vi "FPGA Host-integration mode.vi"() -> ()   [LabVIEW 2015]
uses:
  <vilib>/eio/EIONode/EIONode.xnode
  <vilib>/rvi/eio/common/nirviEmuTemplateMethod_errors.vi
  Globals/Global_Sample per Frame.vi
  Globals/Global Variable_Pixel Clock.vi
panel:
  in  "Number of frames":i32
  out "Samples acquired":u32
  out "Samples per frame_Global":u32
  out "Frame waveform output finish?":bool
  out "Frame acquisition finish?":bool
  out "SubVi Indicator":i32
  out "image data address indicator":u32
  out "Data indicator":u32
  out "Address counter":u32
  out "Pixel clock_indicator":bool
  out "Frame address_indicator":u32
  out "Averaged image displayed? _indicator":bool
  out "Scanning?":bool
  out "loop count":i32
  out "Display_frames done":i32
  out "Averaged data address":u32
  out "Frame imaging data averaged?":bool
  out "Averaged image displayed?":bool
  in  "Kalman gain":fxp<+,16,1>=0.1015625
  in  "Filter gain":fxp<+,16,0>=0.8000030517578125
  in  "Ready to Scan":bool
  out "Pixel clock (Indicator)":bool
  out "Image averaging done?":bool
  in  "Samples per frame control":u32=262144
  out "Data":u32
  out "Galvo signal readed":u32
  out "Request address":u32
  out "Line clock":bool
  in  "Pixel clock_pulse width(tick)":i32
  in  "Resolution":i32
  in  "Pixel pulse_initial delay":i32
  in  "Frame retrace time":u32 caption="Frame retrace time (ms)"
  in  "Num of undershoot":i32
  in  "Elements per line":i32
  in  "Num of elements":u32
  in  "Pixel time (tick)":i32
  out "Write DRAM done?":bool
  in  "Total elements":u32
  out "Frame Galvo signal write done?":bool
  in  "max addr":u32=1024
  in  "Write DRAM enable?":bool
  in  "Write Frame Galvo signal?":bool
  # "Waveform Data Loading"
  # "Photon Counting"
  # "Waveform Generation"
  # "Controller"
  # "Indicator"
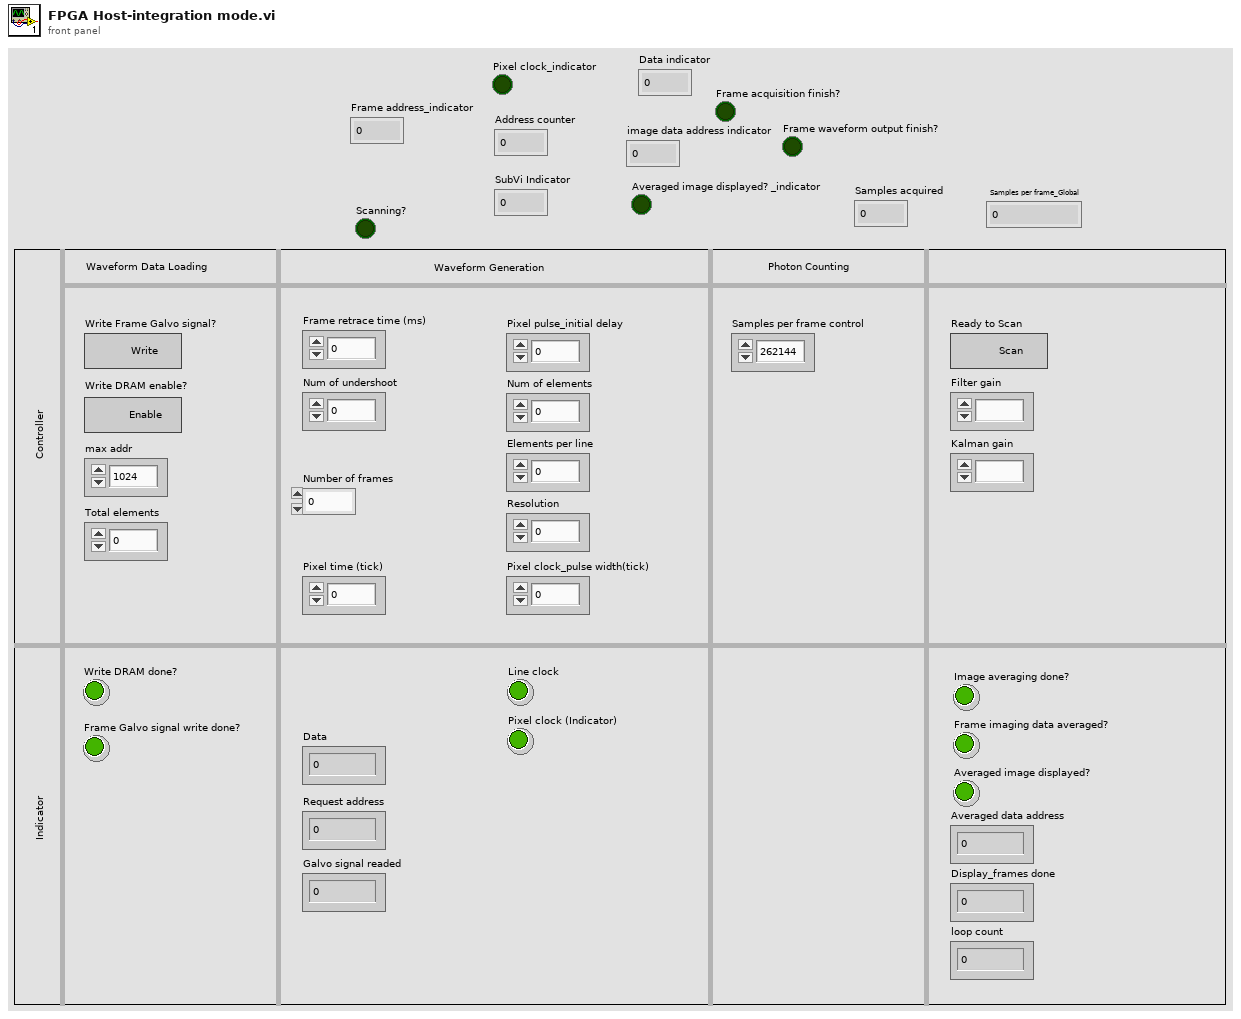
[diagram p1: front panel]
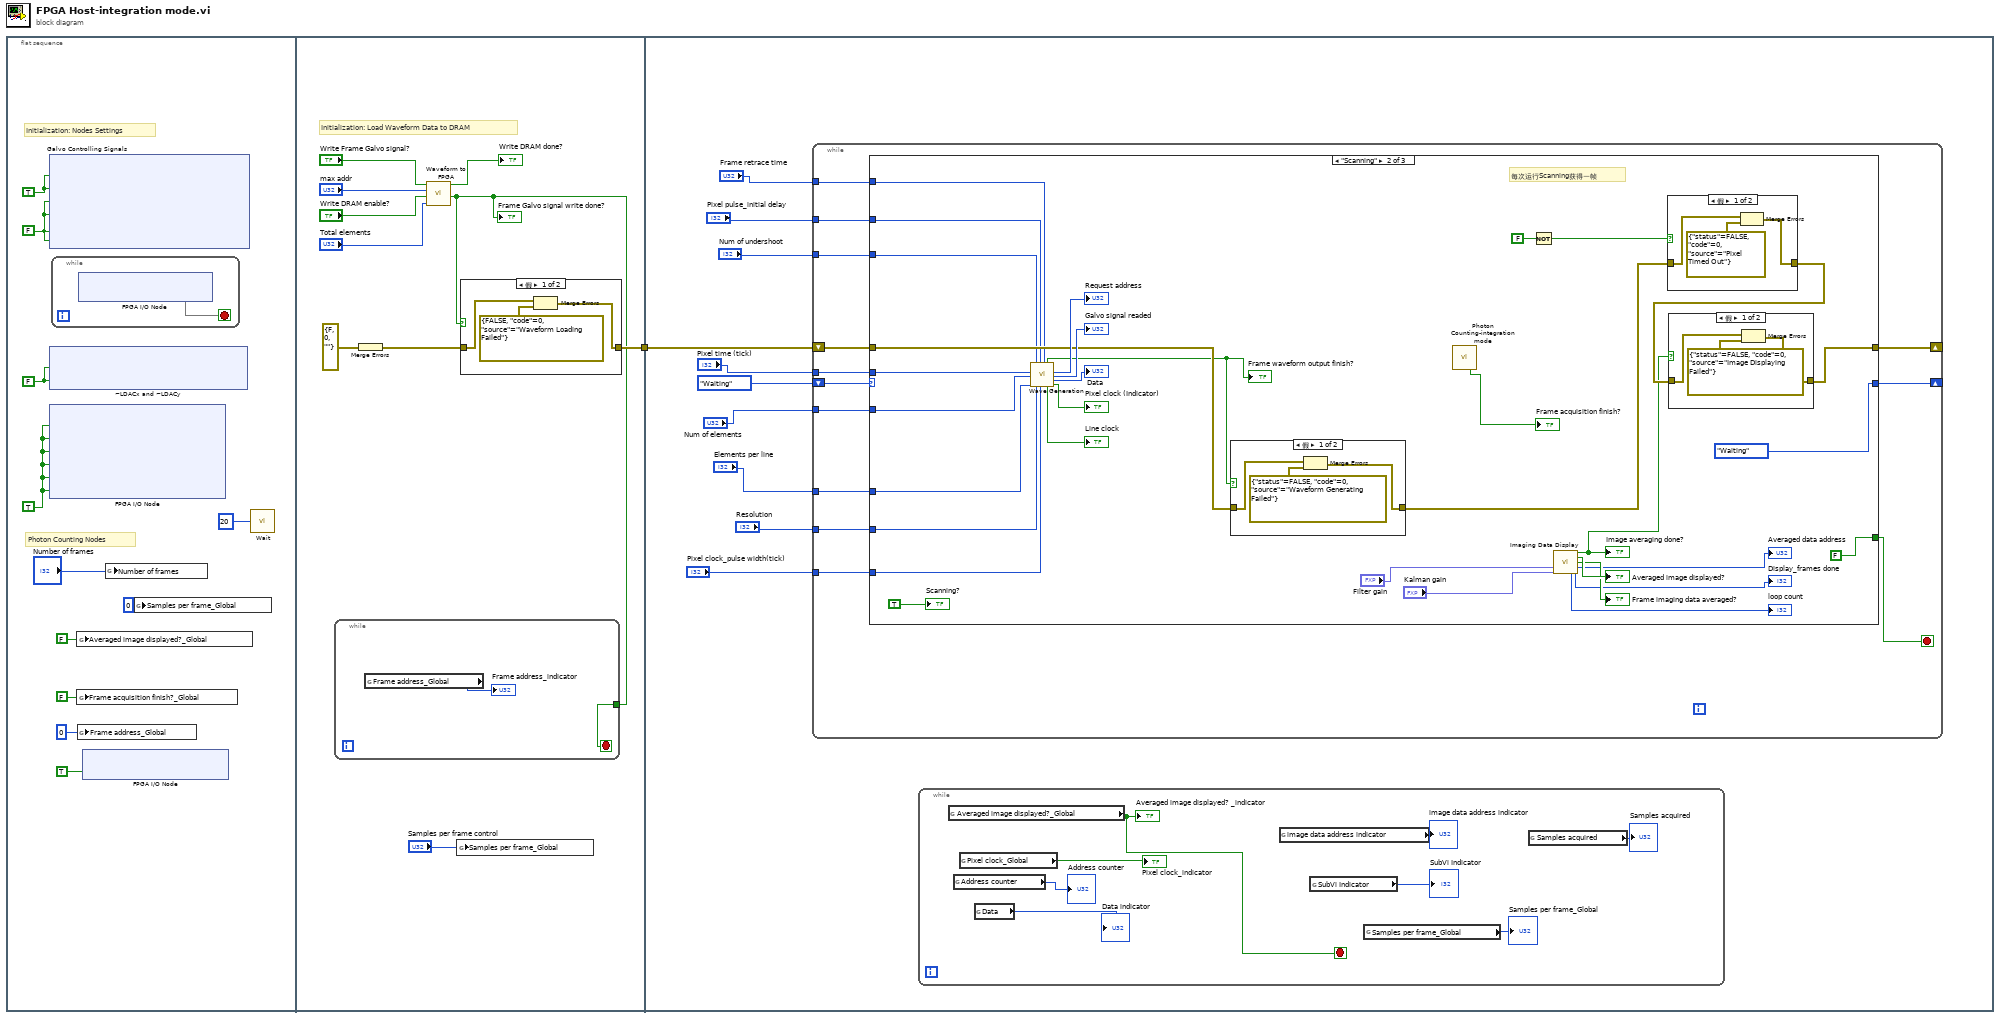
[diagram p0: block diagram]
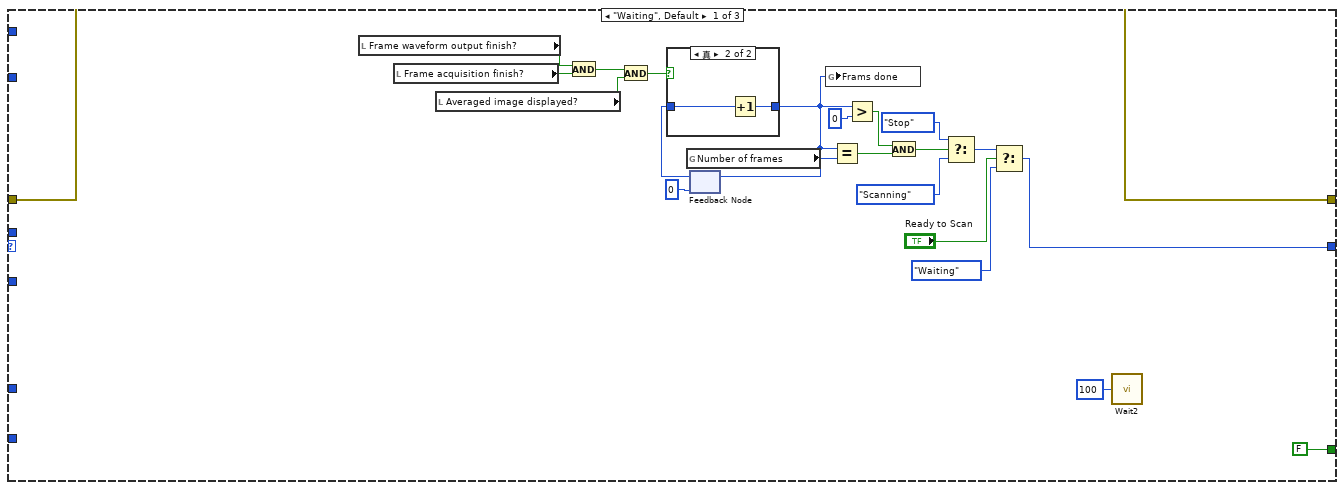
[diagram p3: hidden frame]
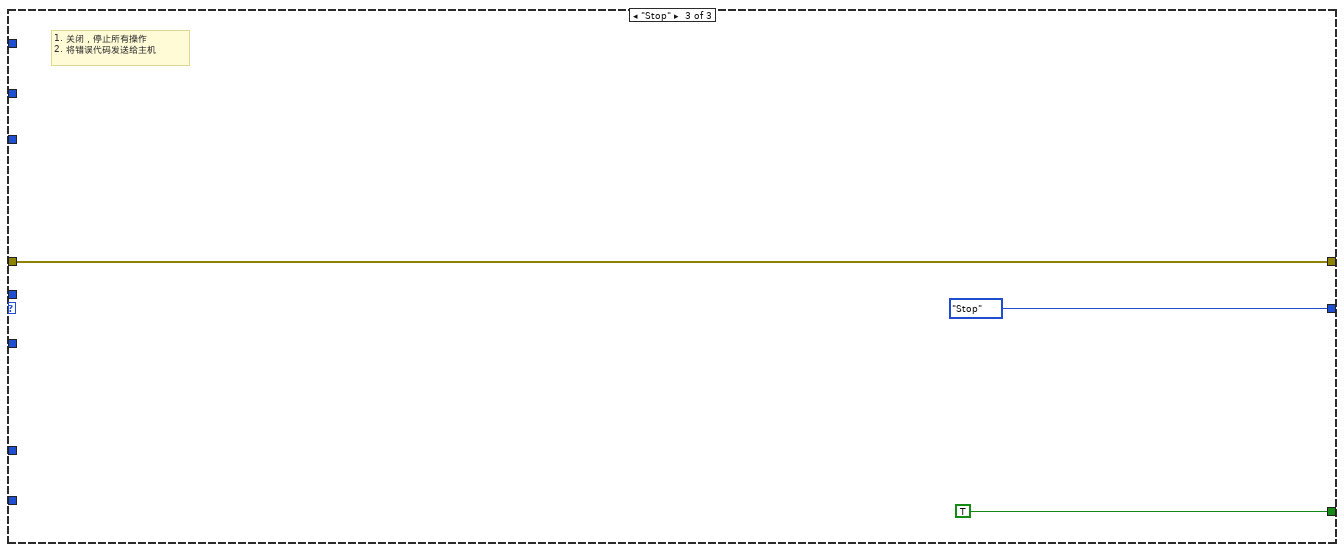
[diagram p8: hidden frame]
diagram:
  n1 = flat-sequence {
    tunnel: [w16] -> w1
    tunnel: w1 -> [w38]
    frame #0 {
      w9 = TRUE ("IO Module\\DDCA_DIO8-15_WE")
      w10 = FALSE ("_LDACx")
      w11 = FALSE ("_CSx")
      w12 = TRUE ("_CLRx")
      # "Photon Counting Nodes"
      # "Initialization: Nodes Settings"
      n2 = xnode "Galvo Controlling Signals"("IO Module\\CLRx(DDCB_DIO0_WRITE)"=w12, "IO Module\\CLRy(DDCB_DIO1_WRITE)"=w12, "IO Module\\CSx(DDCB_DIO2_WRITE)"=w11, "IO Module\\CSy(DDCB_DIO3_WRITE)"=w11, "IO Module\\R_Wx(DDCB_DIO4_WRITE)"=w11, "IO Module\\R_Wy(DDCB_DIO5_WRITE)"=w11) -> ()  [unwired: 6 in, 6 out]
      n3 = xnode "~LDACx and ~LDACy"("IO Module\\LDAx(DDCB_DIO6_WRITE)"=w10, "IO Module\\LDAy(DDCB_DIO7_WRITE)"=w10) -> ()  [unwired: 2 in, 2 out]
      n4 = xnode "FPGA I/O Node"("IO Module\\DDCA_DIO8-15_WE"=w9, "IO Module\\DDCA_DIO16-23_WE"=w9, "IO Module\\DDCB_DIO8-15_WE"=w9, "IO Module\\DDCB_DIO16-23_WE"=w9, "IO Module\\DDCB_DIO0-7_WE"=w9, "IO Module\\DDCB_PFI_WE"=w9) -> ()  [unwired: 6 in, 6 out]
      n5 = while {
        stop <- w13 stop-if-true
        n6 = xnode "FPGA I/O Node"() -> ("IO Module IO Enabled"=w13)  [unwired: 1 in, 1 out]
      }
      n7 = global write "Global_Sample per Frame.vi" "Averaged image displayed?_Global"(FALSE ("Averaged image displayed?")) -> ()
      n8 = global write "Global_Sample per Frame.vi" "Frame acquisition finish?_Global"(FALSE ("Frame acquisition finish?")) -> ()
      n9 = global write "Global_Sample per Frame.vi" "Frame address_Global"(u32 0 ("Frame address")) -> ()
      n10 = xnode "FPGA I/O Node"("IO Module\\DDCA_PFI_WE"=TRUE ("IO Module\\DDCA_DIO8-15_WE")) -> ()  [unwired: 1 in, 1 out]
      n11 = global write "Global_Sample per Frame.vi" "Number of frames"("Number of frames") -> ()
      n12 = global write "Global_Sample per Frame.vi" "Samples per frame_Global"(u32 0 ("Samples per frame_Global")) -> ()
      n13 = call "Wait"("Count(mSec)"=u32 20) -> ()  [unwired: 1 out]
    }
    frame #1 {
      # "Initialization: Load Waveform Data to DRAM"
      n14 = Merge Errors(errorcluster {"status"=FALSE, "code"=0, "source"=""} ("错误输入")) -> (w17:errorcluster)
      n15 = call "Waveform to FPGA.vi"("Write Frame Galvo signal?"="Write Frame Galvo signal?", "max addr"="max addr", "Write DRAM enable?"="Write DRAM enable?", "Total elements"="Total elements") -> ("Write DRAM done?"=→"Write DRAM done?":bool, "Frame Galvo signal write done?"=w15:bool)  [unwired: 5 in]
      "Frame Galvo signal write done?" <- w15
      n16 = while {
        tunnel: w15 -> [w24]
        stop <- w24 stop-if-true
        n17 = global read "Global_Sample per Frame.vi" "Frame address_Global"() -> (→"Frame address_indicator":u32)
      }
      n18 = global write "Global_Sample per Frame.vi" "Samples per frame_Global"("Samples per frame control") -> ()
      n19 = case shown="假" w15 {
        tunnel: w17 -> [w28 w29]
        tunnel: [w26 w29] -> w16
        frame False {
          n20 = Merge Errors(w28, cluster{bool, "code":i32, "source":string} {FALSE, "code"=0, "source"="Waveform Loading Failed"} ("错误输入")) -> (w26:errorcluster)
        }
        frame True {
        }
      }
    }
    frame #2 {
      n21 = while {
        shift-right: [w59] -> _
        shift-left: enum16{"Waiting", "Scanning", "Stop"}."Waiting" -> [w60]
        shift-right: [w57] -> _
        shift-left: w38 -> [w58]
        tunnel: "Frame retrace time" -> [w56]
        tunnel: "Pixel pulse_initial delay" -> [w55]
        tunnel: "Num of undershoot" -> [w54]
        tunnel: "Pixel time (tick)" -> [w53]
        tunnel: "Num of elements" -> [w52]
        tunnel: "Elements per line" -> [w51]
        tunnel: "Resolution" -> [w50]
        tunnel: "Pixel clock_pulse width(tick)" -> [w49]
        stop <- w48 stop-if-true
        n22 = case shown="\"Scanning\"" w60 {
          tunnel: [w81 enum16{"Waiting", "Scanning", "Stop"}."Waiting" enum16{"Waiting", "Scanning", "Stop"}."Stop"] -> w59
          tunnel: w58 -> [w82 w112 w132]
          tunnel: [w82 w106 w132] -> w57
          tunnel: w56 -> [_ w99 _]
          tunnel: w55 -> [_ w98 _]
          tunnel: w54 -> [_ w97 _]
          tunnel: w53 -> [_ w96 _]
          tunnel: w52 -> [_ w95 _]
          tunnel: w51 -> [_ w94 _]
          tunnel: w50 -> [_ w93 _]
          tunnel: w49 -> [_ w92 _]
          tunnel: [FALSE FALSE TRUE] -> w48
          frame "Waiting", Default {
            n23 = local read "Frame waveform output finish?"() -> (w72:bool)
            n24 = local read "Frame acquisition finish?"() -> (w73:bool)
            n25 = local read "Averaged image displayed?"() -> (w74:bool)
            n26 = And(x=w72, y=w73) -> (x .and. y?=w75:bool)
            n27 = And(x=w75, y=w74) -> (x .and. y?=w77:bool)
            n28 = global read "Global_Sample per Frame.vi" "Number of frames"() -> (w67:i32)
            n29 = feedback #1(0) -> (w76:i32)
            n30 = case shown="真" w77 {
              tunnel: w76 -> [w83 w84]
              tunnel: [w83 w85] -> w66
              frame False {
              }
              frame True {
                n31 = Increment(x=w84) -> (x+1=w85:i32)
              }
            }
            n32 = feedback-in #1(w66) -> ()
            n33 = global write "Global_Sample per Frame.vi" "Frams done"(w66) -> ()
            n34 = Equal?(x=w66, y=w67) -> (x = y?=w63:bool)
            n35 = Greater?(x=w66, y=0) -> (0:w64:bool)
            n36 = And(x=w64, y=w63) -> (x .and. y?=w62:bool)
            n37 = Select(t=enum16{"Waiting", "Scanning", "Stop"}."Stop", s=w62, f=enum16{"Waiting", "Scanning", "Stop"}."Scanning") -> (s? t:f=w68:enum16{"Waiting", "Scanning", "Stop"})
            n38 = Select(t=w68, s="Ready to Scan", f=enum16{"Waiting", "Scanning", "Stop"}."Waiting") -> (s? t:f=w81:enum16{"Waiting", "Scanning", "Stop"})
            n39 = call "Wait2"("Count(mSec)"=u32 100) -> ()  [unwired: 1 out]
          }
          frame "Scanning" {
            # "每次运行Scanning获得一帧"
            n40 = call "Wave Generation.vi"("Pixel time (tick)"=w96, "Num of elements"=w95, "Elements per line"=w94, "Num of undershoot"=w97, "Resolution"=w93, "Pixel pulse_initial delay"=w98, "Pixel clock_pulse width(tick)"=w92, "Frame retrace time"=w99) -> ("Frame waveform output finish?"=w91:bool, "Line clock"=→"Line clock":bool, "Request address"=→"Request address":u32, "Galvo signal readed"=→"Galvo signal readed":u32, "Data"=→"Data":u32, "Pixel clock"=→"Pixel clock (Indicator)":bool)  [unwired: 6 in]
            "Frame waveform output finish?" <- w91
            n41 = case shown="假" w91 {
              tunnel: w112 -> [w128 w129]
              tunnel: [w126 w129] -> w111
              frame False {
                n42 = Merge Errors(w128, errorcluster {"status"=FALSE, "code"=0, "source"="Waveform Generating Failed"} ("错误输入")) -> (w126:errorcluster)
              }
              frame True {
              }
            }
            n43 = call "Photon Counting-integration mode.vi"() -> ("Frame acquisition finish?"=→"Frame acquisition finish?":bool)  [unwired: 19 in]
            n44 = Not(x=FALSE) -> (.not. x?=w110:bool)
            n45 = call "Imaging Data Display.vi"("Filter gain"="Filter gain", "Kalman gain"="Kalman gain") -> ("Image averaging done?"=w108:bool, "Averaged image displayed?"=→"Averaged image displayed?":bool, "Frame imaging data Averaged?"=→"Frame imaging data averaged?":bool, "Averaged data address"=→"Averaged data address":u32, "loop count"=→"loop count":i32, "Display_frames done"=→"Display_frames done":i32)  [unwired: 8 in]
            "Image averaging done?" <- w108
            n46 = case shown="假" w110 {
              tunnel: w111 -> [w124 w125]
              tunnel: [w122 w125] -> w109
              frame False {
                n47 = Merge Errors(w124, errorcluster {"status"=FALSE, "code"=0, "source"="Pixel Timed Out"} ("错误输入")) -> (w122:errorcluster)
              }
              frame True {
              }
            }
            n48 = case shown="假" w108 {
              tunnel: w109 -> [w120 w121]
              tunnel: [w118 w121] -> w106
              frame False {
                n49 = Merge Errors(w120, errorcluster {"status"=FALSE, "code"=0, "source"="Image Displaying Failed"} ("错误输入")) -> (w118:errorcluster)
              }
              frame True {
              }
            }
            "Scanning?" <- TRUE
          }
          frame "Stop" {
            # "1. 关闭，停止所有操作\n2. 将错误代码发送给主机"
          }
        }
      }
      n50 = while {
        stop <- w40 stop-if-true
        n51 = global read "Global_Sample per Frame.vi" "Averaged image displayed?_Global"() -> (w40:bool)
        "Averaged image displayed? _indicator" <- w40
        n52 = global read "Global_Sample per Frame.vi" "Address counter"() -> (→"Address counter":u32)
        n53 = global read "Global Variable_Pixel Clock.vi" "Pixel clock_Global"() -> (→"Pixel clock_indicator":bool)
        n54 = global read "Global_Sample per Frame.vi" "Data"() -> (→"Data indicator":u32)
        n55 = global read "Global_Sample per Frame.vi" "image data address indicator"() -> (→"image data address indicator":u32)
        n56 = global read "Global_Sample per Frame.vi" "SubVi Indicator"() -> (→"SubVi Indicator":i32)
        n57 = global read "Global_Sample per Frame.vi" "Samples per frame_Global"() -> (→"Samples per frame_Global":u32)
        n58 = global read "Global_Sample per Frame.vi" "Samples acquired"() -> (→"Samples acquired":u32)
      }
    }
  }
